vi "ExportToWord.vi"(11 "DataForAnalysis":T1(array[cluster]) {"Eff" scale=0.0..30.0; "JVmetrics" format="%#_4g"}) -> ()   [LabVIEW 2020]
uses:
  <vilib>/Utility/NIReport.llb/NI_report.lvclass
  <vilib>/addons/_office/word.llb/Word Easy Table (num).vi
  <vilib>/Utility/NIReport.llb/Append Report Text (str wrap).vi
  <vilib>/addons/_office/_exclsub.llb/font.ctl
panel:
  in  "Plot Color 2":u32[](array[colorbox])=[16711686]
  in  "Plot Area Color 2":u32(colorbox)=16777215
  in  "Axis Font 2":T2={"font style"="", "bold"=FALSE, "italic"=FALSE, "underline"=FALSE, "size"=10.0, "color"=4278190080} {"size" format="%.2f"}
  in  "Y Axis Configuration 2":T3={"Autoscale"=TRUE, "min"=0.0, "max"=0.0, "scale type"=-4132} {"scale type" items=["xlScaleLinear"=-4132, "xlScaleLogarithmic"=-4133]; "max" format="%.2f"; "min" format="%.2f"}
  in  "X Axis Configuration 2":T4={"autoscale"=TRUE, "min"=0.0, "max"=0.0, "scale type"=-4132} {"scale type" items=["xlScaleLinear"=-4132, "xlScaleLogarithmic"=-4133]; "max" format="%.2f"; "min" format="%.2f"}
  in  "graph title (\"\") 2":string="Transient data"
  in  "yAxisT 2":string="Power (mW/cm2)"
  in  "XAxisT 2":string="time (s)"
  out "transposed array":dbl[][](array[numeric])=[[1.0, 0.0], [0.0, 0.0], [0.0, 0.0], [1.0, 0.0], [0.0, 0.0], [1.0, 1.0]]
  in  "column headers":string[](array[string])=["1st scan", "2nd scan"]
  in  "indent and spacing":T5 {"at" format="%.2f"; "after" format="%.2f"; "before" format="%.2f"; "by" format="%.2f"; "right" format="%.2f"; "left" format="%.2f"}
  in  "line and page breaks":T6={"widow/orphan ctrl"=2, "Keeps lines together"=0, "keep with next"=0, "page break before"=0, "suppress line numbers"=0, "don't hyphenate"=0} {"don't hyphenate" items=["Unchanged", "No", "Yes"]; "suppress line numbers" items=["Unchanged", "No", "Yes"]; "page break before" items=["Unchanged", "No", "Yes"]; "keep with next" items=["Unchanged", "No", "Yes"]; "Keeps lines together" items=["Unchanged", "No", "Yes"]; "widow/orphan ctrl" items=["Unchanged", "No", "Yes"]}
  in  "auto format (none)":i32=-1
  in  "font":T7={"font name"="", "font size"=10.0, "bold"=2, "italic"=0, "underline"=0, "strike through"=0, "font color"=16777216} {"font size" format="%0.2f"; "strike through" items=["Unchanged", "Yes", "No"]; "underline" items=["Unchanged", "Yes", "No"]; "italic" items=["Unchanged", "Yes", "No"]; "bold" items=["Unchanged", "Yes", "No"]}
  in  "HeaderJVMetrics":string[](array[string])=["Voc (V)", "Jsc (mA/cm2)", "FF", "P (mW/cm2)", "Hyst P1/P2", "scan rate (mV/s)", "intensity (suns)", "temperature (C)"]
  in  "XAxisT":string="Voltage (V)"
  in  "yAxisT":string="Current Density (mA/cm2)"
  in  "graph title (\"\")":string="JV data"
  in  "X Axis Configuration":T4={"autoscale"=TRUE, "min"=0.0, "max"=0.0, "scale type"=-4132} {"scale type" items=["xlScaleLinear"=-4132, "xlScaleLogarithmic"=-4133]; "max" format="%.2f"; "min" format="%.2f"}
  in  "Y Axis Configuration":T3={"Autoscale"=TRUE, "min"=0.0, "max"=0.0, "scale type"=-4132} {"scale type" items=["xlScaleLinear"=-4132, "xlScaleLogarithmic"=-4133]; "max" format="%.2f"; "min" format="%.2f"}
  in  "Axis Font":T2={"font style"="", "bold"=FALSE, "italic"=FALSE, "underline"=FALSE, "size"=10.0, "color"=4278190080} {"size" format="%.2f"}
  in  "Plot Area Color":u32(colorbox)=16777215
  in  "Plot Color":u32[](array[colorbox])=[16860]
  # "indentation"
  # "spacing"
  # "pagination"
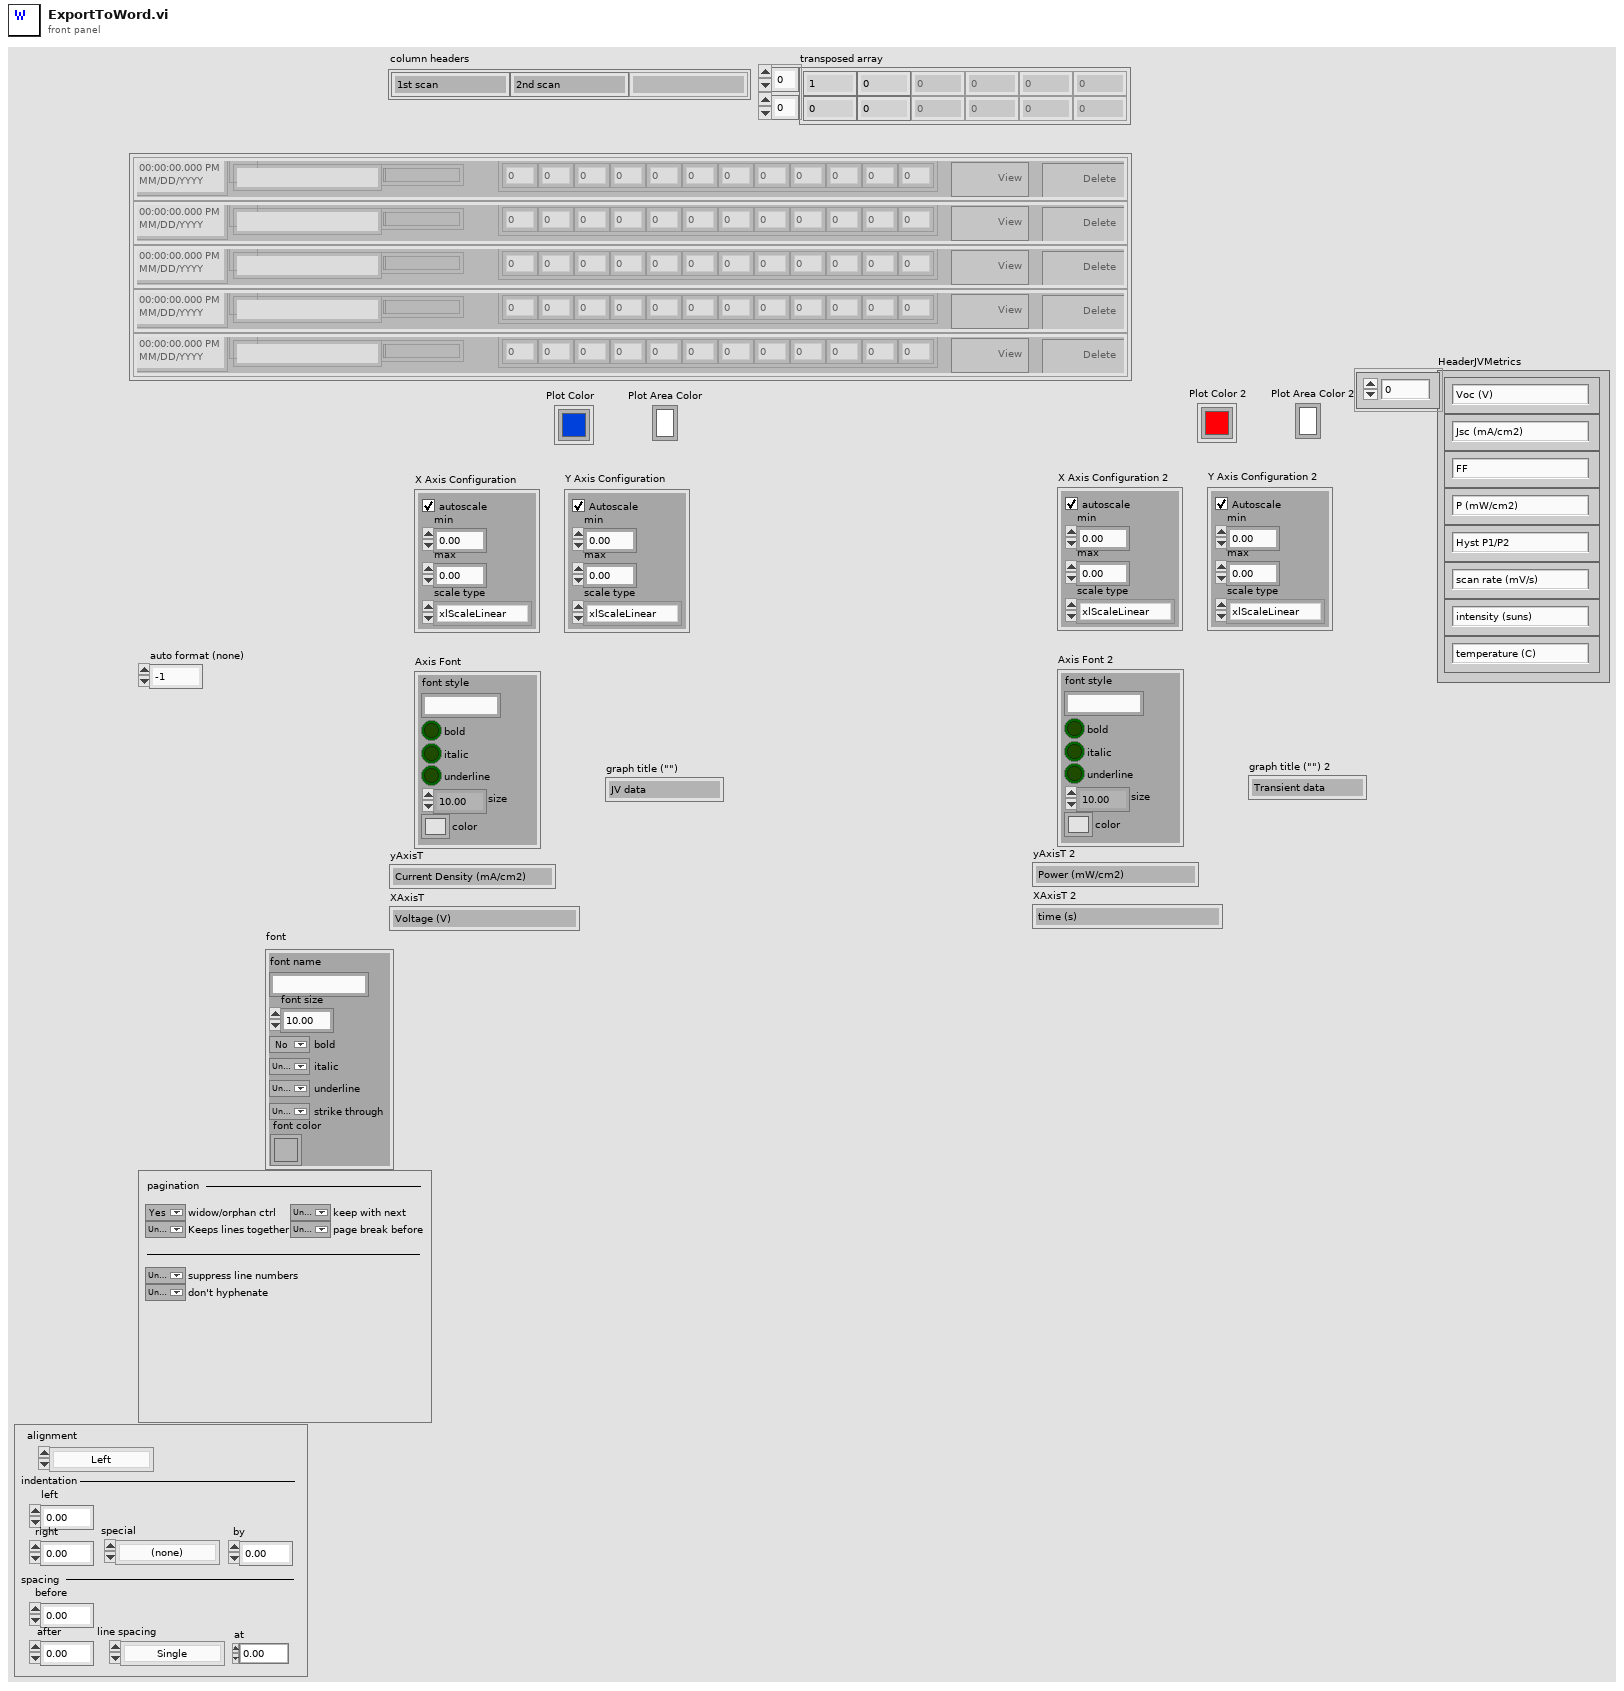
[diagram p1: front panel]
types:
  T1 = cluster{"JVData":dbl[][], "JVmetrics":dbl[], "TransientData":dbl[][], "TimeMeasured":timestamp, "Name":string, "Delete":bool, "Eff":u8, "ViewJV":bool}[]
  T2 = cluster{"font style":string, "bold":bool, "italic":bool, "underline":bool, "size":sgl, "color":u32}
  T3 = cluster{"Autoscale":bool, "min":dbl, "max":dbl, "scale type":i32}
  T4 = cluster{"autoscale":bool, "min":dbl, "max":dbl, "scale type":i32}
  T5 = cluster{"alignment":enum16{"Left", "Centered", "Right", "Justify"}, "left":dbl, "right":dbl, "special":enum16{"(none)", "First line", "Hanging"}, "by":dbl, "before":dbl, "after":dbl, "line spacing":enum16{"Single", "1,5 lines", "Double", "At least", "Exactly", "Multiple"}, "at":dbl}
  T6 = cluster{"widow/orphan ctrl":u16, "Keeps lines together":u16, "keep with next":u16, "page break before":u16, "suppress line numbers":u16, "don't hyphenate":u16}
  T7 = typedef "NI_ReportGenerationToolkit.lvlib/font.ctl" = cluster{"font name":string, "font size":dbl, "bold":u16, "italic":u16, "underline":u16, "strike through":u16, "font color":u32}
  T8 = enum16{"Standard Report", "HTML", "Word", "Excel"}
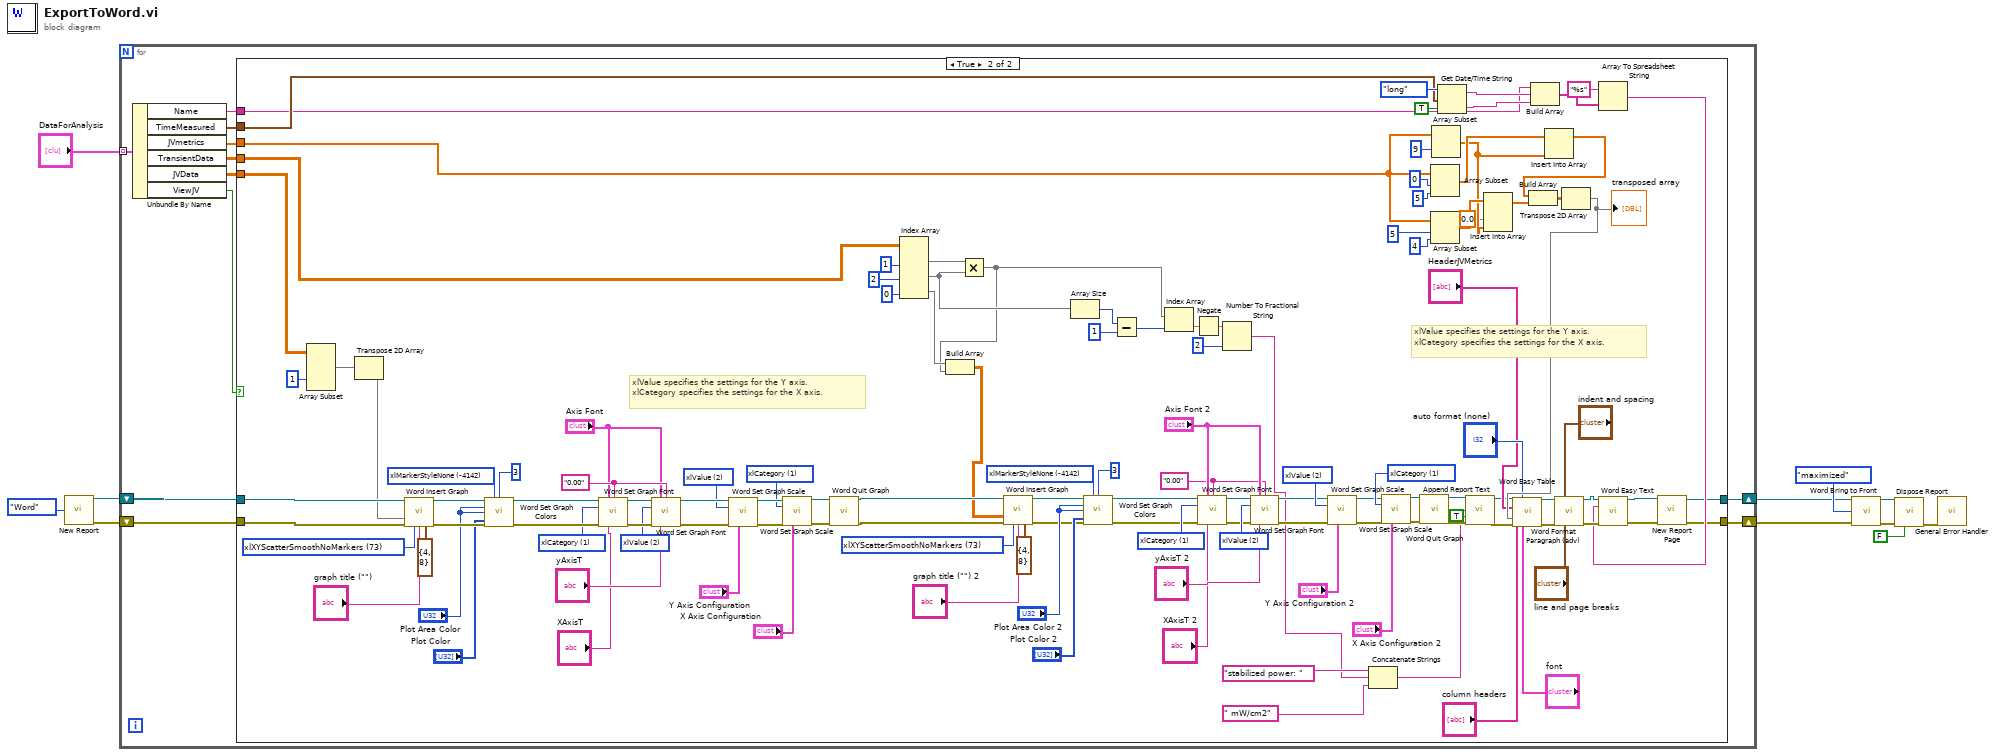
[diagram p0: block diagram]
diagram:
  n1 = call <vilib>:"New Report.vi"("report type"=T8."Word") -> ("report out"=w10:refnum<class "NI_report.lvclass">, "error out"=w11:errorcluster)  [unwired: 13 in]
  n2 = for {
    shift-right: [w17] -> w3
    shift-left: w11 -> [w22]
    shift-right: [w16] -> w2
    shift-left: w10 -> [w21]
    tunnel: "DataForAnalysis" -> [w15] mode=indexing
    n3 = Unbundle By Name(w15) -> ("Name"=w19:string, "TimeMeasured"=w20:timestamp, "JVmetrics"=w18:dbl[], "TransientData"=w13:dbl[][], "JVData"=w14:dbl[][], "ViewJV"=w12:bool)
    n4 = case shown="True" w12 {
      tunnel: w22 -> [w23 w151]
      tunnel: w21 -> [w24 w150]
      tunnel: w20 -> [_ w119]
      tunnel: w19 -> [_ w104]
      tunnel: w18 -> [_ w98]
      tunnel: [w23 w60] -> w17
      tunnel: [w24 w59] -> w16
      tunnel: w14 -> [_ w35]
      tunnel: w13 -> [_ w40]
      frame False {
      }
      frame True {
        w89 = "0.00" ("number format (general)")
        w86 = 1 items=["xlCategory"=1, "xlSeriesAxis"=3, "xlValue"=2] ("axis type")
        w83 = 2 items=["xlCategory"=1, "xlSeriesAxis"=3, "xlValue"=2] ("axis type")
        w80 = 2 items=["xlCategory"=1, "xlSeriesAxis"=3, "xlValue"=2] ("axis type")
        w77 = 1 items=["xlCategory"=1, "xlSeriesAxis"=3, "xlValue"=2] ("axis type")
        w74 = -4142 items=["xlMarkerStyleAutomatic"=-4105, "xlMarkerStyleCircle"=8, "xlMarkerStyleDash"=-4115, "xlMarkerStyleDiamond"=2, "xlMarkerStyleDot"=-4118, "xlMarkerStyleNone"=-4142, "xlMarkerStylePicture"=-4147, "xlMarkerStylePlus"=9, "xlMarkerStyleSquare"=1, "xlMarkerStyleStar"=5, "xlMarkerStyleTriangle"=3, "xlMarkerStyleX"=-4168] ("marker style")
        w69 = 73 items=["xlColumnClustered"=51, "xlColumnStacked"=52, "xlColumnStacked100"=53, "xl3DColumnClustered"=54, "xl3DColumnStacked"=55, "xl3DColumnStacked100"=56, "xlBarClustered"=57, "xlBarStacked"=58, "xlBarStacked100"=59, "xl3DBarClustered"=60, "xl3DBarStacked"=61, "xl3DBarStacked100"=62, "xlLineStacked"=63, "xlLineStacked100"=64, "xlLineMarkers"=65, "xlLineMarkersStacked"=66, "xlLineMarkersStacked100"=67, "xlPieOfPie"=68, "xlPieExploded"=69, "xl3DPieExploded"=70, "xlBarOfPie"=71, "xlXYScatterSmooth"=72, "xlXYScatterSmoothNoMarkers"=73, "xlXYScatterLines"=74, "xlXYScatterLinesNoMarkers"=75, "xlAreaStacked"=76, "xlAreaStacked100"=77, "xl3DAreaStacked"=78, "xl3DAreaStacked100"=79, "xlDoughnutExploded"=80, "xlRadarMarkers"=81, "xlRadarFilled"=82, "xlSurface"=83, "xlSurfaceWireframe"=84, "xlSurfaceTopView"=85, "xlSurfaceTopViewWireframe"=86, "xlBubble"=15, "xlBubble3DEffect"=87, "xlStockHLC"=88, "xlStockOHLC"=89, "xlStockVHLC"=90, "xlStockVOHLC"=91, "xlCylinderColClustered"=92, "xlCylinderColStacked"=93, "xlCylinderColStacked100"=94, "xlCylinderBarClustered"=95, "xlCylinderBarStacked"=96, "xlCylinderBarStacked100"=97, "xlCylinderCol"=98, "xlConeColClustered"=99, "xlConeColStacked"=100, "xlConeColStacked100"=101, "xlConeBarClustered"=102, "xlConeBarStacked"=103, "xlConeBarStacked100"=104, "xlConeCol"=105, "xlPyramidColClustered"=106, "xlPyramidColStacked"=107, "xlPyramidColStacked100"=108, "xlPyramidBarClustered"=109, "xlPyramidBarStacked"=110, "xlPyramidBarStacked100"=111, "xlPyramidCol"=112, "xl3DColumn"=-4100, "xlLine"=4, "xl3DLine"=-4101, "xl3DPie"=-4102, "xlPie"=5, "xlXYScatter"=-4169, "xl3DArea"=-4098, "xlArea"=1, "xlDoughnut"=-4120, "xlRadar"=-4151] ("chart type")
        w129 = "0.00" ("number format (general)")
        w132 = 1 items=["xlCategory"=1, "xlSeriesAxis"=3, "xlValue"=2] ("axis type")
        w135 = 2 items=["xlCategory"=1, "xlSeriesAxis"=3, "xlValue"=2] ("axis type")
        w138 = 2 items=["xlCategory"=1, "xlSeriesAxis"=3, "xlValue"=2] ("axis type")
        w141 = 1 items=["xlCategory"=1, "xlSeriesAxis"=3, "xlValue"=2] ("axis type")
        w144 = -4142 items=["xlMarkerStyleAutomatic"=-4105, "xlMarkerStyleCircle"=8, "xlMarkerStyleDash"=-4115, "xlMarkerStyleDiamond"=2, "xlMarkerStyleDot"=-4118, "xlMarkerStyleNone"=-4142, "xlMarkerStylePicture"=-4147, "xlMarkerStylePlus"=9, "xlMarkerStyleSquare"=1, "xlMarkerStyleStar"=5, "xlMarkerStyleTriangle"=3, "xlMarkerStyleX"=-4168] ("marker style")
        w149 = 73 items=["xlColumnClustered"=51, "xlColumnStacked"=52, "xlColumnStacked100"=53, "xl3DColumnClustered"=54, "xl3DColumnStacked"=55, "xl3DColumnStacked100"=56, "xlBarClustered"=57, "xlBarStacked"=58, "xlBarStacked100"=59, "xl3DBarClustered"=60, "xl3DBarStacked"=61, "xl3DBarStacked100"=62, "xlLineStacked"=63, "xlLineStacked100"=64, "xlLineMarkers"=65, "xlLineMarkersStacked"=66, "xlLineMarkersStacked100"=67, "xlPieOfPie"=68, "xlPieExploded"=69, "xl3DPieExploded"=70, "xlBarOfPie"=71, "xlXYScatterSmooth"=72, "xlXYScatterSmoothNoMarkers"=73, "xlXYScatterLines"=74, "xlXYScatterLinesNoMarkers"=75, "xlAreaStacked"=76, "xlAreaStacked100"=77, "xl3DAreaStacked"=78, "xl3DAreaStacked100"=79, "xlDoughnutExploded"=80, "xlRadarMarkers"=81, "xlRadarFilled"=82, "xlSurface"=83, "xlSurfaceWireframe"=84, "xlSurfaceTopView"=85, "xlSurfaceTopViewWireframe"=86, "xlBubble"=15, "xlBubble3DEffect"=87, "xlStockHLC"=88, "xlStockOHLC"=89, "xlStockVHLC"=90, "xlStockVOHLC"=91, "xlCylinderColClustered"=92, "xlCylinderColStacked"=93, "xlCylinderColStacked100"=94, "xlCylinderBarClustered"=95, "xlCylinderBarStacked"=96, "xlCylinderBarStacked100"=97, "xlCylinderCol"=98, "xlConeColClustered"=99, "xlConeColStacked"=100, "xlConeColStacked100"=101, "xlConeBarClustered"=102, "xlConeBarStacked"=103, "xlConeBarStacked100"=104, "xlConeCol"=105, "xlPyramidColClustered"=106, "xlPyramidColStacked"=107, "xlPyramidColStacked100"=108, "xlPyramidBarClustered"=109, "xlPyramidBarStacked"=110, "xlPyramidBarStacked100"=111, "xlPyramidCol"=112, "xl3DColumn"=-4100, "xlLine"=4, "xl3DLine"=-4101, "xl3DPie"=-4102, "xlPie"=5, "xlXYScatter"=-4169, "xl3DArea"=-4098, "xlArea"=1, "xlDoughnut"=-4120, "xlRadar"=-4151] ("chart type")
        # "xlValue specifies the settings for the Y axis. xlCategory specifies the settings for the X axis."
        # "xlValue specifies the settings for the Y axis. xlCategory specifies the settings for the X axis."
        n5 = Array Subset(array=w35, index (col)=1 ("index")) -> (w32:dbl[][])  [unwired: 3 in]
        n6 = Transpose 2D Array(2D array=w32) -> (transposed array=w33:dbl[][])
        n7 = call <vilib>:"Word Insert Graph.vi"("report in"=w150, "data"=w33, "error in (no error)"=w151, "graph type (col clustered)"=w149, "graph title (\"\")"="graph title (\"\")", "graph size (5, 5)"=cluster{"Height":i32, "Width":i32} {"Height"=4, "Width"=8} ("chart size")) -> ("report out"=w146:refnum<class "NI_report.lvclass">, "error out"=w147:errorcluster)  [unwired: 6 in, 2 out]
        n8 = call <vilib>:"Word Set Graph Colors.vi"("report in"=w146, "marker style (none)"=w144, "weight (1)"=i16 3 ("weight"), "plot area color (w)"="Plot Area Color", "graph area color (w)"="Plot Area Color", "error in (no error)"=w147, "plot colors"="Plot Color") -> ("report out"=w142:refnum<class "NI_report.lvclass">, "error out"=w143:errorcluster)  [unwired: 7 in]
        n9 = call <vilib>:"Word Set Graph Font.vi"("report in"=w142, "axis font"="Axis Font", "number format (general)"=w129, "axis type (category)"=w141, "error in (no error)"=w143, "title (\"\")"="XAxisT") -> ("report out"=w139:refnum<class "NI_report.lvclass">, "error out"=w140:errorcluster)  [unwired: 8 in]
        n10 = call <vilib>:"Word Set Graph Font.vi"("report in"=w139, "axis font"="Axis Font", "number format (general)"=w129, "axis type (category)"=w138, "error in (no error)"=w140, "title (\"\")"="yAxisT") -> ("report out"=w136:refnum<class "NI_report.lvclass">, "error out"=w137:errorcluster)  [unwired: 8 in]
        n11 = call <vilib>:"Word Set Graph Scale.vi"("report in"=w136, "axis type (xlCategory)"=w135, "error in (no error)"=w137, "axis config"="Y Axis Configuration") -> ("report out"=w133:refnum<class "NI_report.lvclass">, "error out"=w134:errorcluster)  [unwired: 10 in]
        n12 = call <vilib>:"Word Set Graph Scale.vi"("report in"=w133, "axis type (xlCategory)"=w132, "error in (no error)"=w134, "axis config"="X Axis Configuration") -> ("report out"=w131:refnum<class "NI_report.lvclass">, "error out"=w130:errorcluster)  [unwired: 10 in]
        n13 = call <vilib>:"Word Quit Graph.vi"("report in"=w131, "error in (no error)"=w130) -> ("report out"=w68:refnum<class "NI_report.lvclass">, "error out"=w67:errorcluster)  [unwired: 12 in]
        n14 = Index Array(array=w40, index (col) #1=1 ("disabled index (col)"), index (col) #2=2 ("index (col)"), index (col) #3=0 ("index (col)")) -> (element #1=w44:dbl[], element #2=w43:dbl[], element #3=w38:dbl[])  [unwired: 3 in]
        n15 = Multiply(x=w44, y=w43) -> (x*y=w37:dbl[])
        n16 = Build Array(w38, w37) -> (w36:dbl[][])
        n17 = call <vilib>:"Word Insert Graph.vi"("report in"=w68, "data"=w36, "error in (no error)"=w67, "graph type (col clustered)"=w69, "graph title (\"\")"="graph title (\"\") 2", "graph size (5, 5)"=cluster{"Height":i32, "Width":i32} {"Height"=4, "Width"=8} ("chart size")) -> ("report out"=w72:refnum<class "NI_report.lvclass">, "error out"=w71:errorcluster)  [unwired: 6 in, 2 out]
        n18 = Array Size(array=w43) -> (size(s)=w48:i32)
        n19 = call <vilib>:"Word Set Graph Colors.vi"("report in"=w72, "marker style (none)"=w74, "weight (1)"=i16 3 ("weight"), "plot area color (w)"="Plot Area Color 2", "graph area color (w)"="Plot Area Color 2", "error in (no error)"=w71, "plot colors"="Plot Color 2") -> ("report out"=w76:refnum<class "NI_report.lvclass">, "error out"=w75:errorcluster)  [unwired: 7 in]
        n20 = Subtract(x=w48, y=1) -> (x-y=w49:i32)
        n21 = Index Array(array=w37, index=w49) -> (element=w30:dbl)
        n22 = Negate(x=w30) -> (-x=w31:dbl)
        n23 = call <vilib>:"Word Set Graph Font.vi"("report in"=w76, "axis font"="Axis Font 2", "number format (general)"=w89, "axis type (category)"=w77, "error in (no error)"=w75, "title (\"\")"="XAxisT 2") -> ("report out"=w79:refnum<class "NI_report.lvclass">, "error out"=w78:errorcluster)  [unwired: 8 in]
        n24 = Number To Fractional String(number=w31, precision (6)=i16 2) -> (F-format string=w42:string)  [unwired: 2 in]
        n25 = call <vilib>:"Word Set Graph Font.vi"("report in"=w79, "axis font"="Axis Font 2", "number format (general)"=w89, "axis type (category)"=w80, "error in (no error)"=w78, "title (\"\")"="yAxisT 2") -> ("report out"=w82:refnum<class "NI_report.lvclass">, "error out"=w81:errorcluster)  [unwired: 8 in]
        n26 = call <vilib>:"Word Set Graph Scale.vi"("report in"=w82, "axis type (xlCategory)"=w83, "error in (no error)"=w81, "axis config"="Y Axis Configuration 2") -> ("report out"=w85:refnum<class "NI_report.lvclass">, "error out"=w84:errorcluster)  [unwired: 10 in]
        n27 = Concatenate Strings("stabilized power: ", w42, " mW/cm2") -> (w52:string)
        n28 = call <vilib>:"Word Set Graph Scale.vi"("report in"=w85, "axis type (xlCategory)"=w86, "error in (no error)"=w84, "axis config"="X Axis Configuration 2") -> ("report out"=w87:refnum<class "NI_report.lvclass">, "error out"=w88:errorcluster)  [unwired: 10 in]
        n29 = call <vilib>:"Word Quit Graph.vi"("report in"=w87, "error in (no error)"=w88) -> ("report out"=w57:refnum<class "NI_report.lvclass">, "error out"=w54:errorcluster)  [unwired: 12 in]
        n30 = Array Subset(array=w98, index=0, length=5) -> (w97:dbl[])
        n31 = Array Subset(array=w98, index=5 ("length"), length=4) -> (w27:dbl[])
        n32 = Array Subset(array=w98, index=9 ("length")) -> (w26:dbl[])  [unwired: 1 in]
        n33 = Get Date/Time String(date format (0)=enum16{"short", "long", "abbreviated"}."long", seconds (now)=w119, want seconds? (F)=TRUE) -> (date string=w118:string, time string=w120:string)
        n34 = call-poly <vilib>:"Append Report Text.vi"("report in"=w57, "text"=w52, "append on new line? (F)"=TRUE, "error in (no error)"=w54) -> ("report out"=w56:refnum<class "NI_report.lvclass">, "error out"=w55:errorcluster)  [unwired: 8 in, 2 out]
        n35 = Insert Into Array(array=w27, new element #1=0.0 ("new element/subarray"), new element #2=w26) -> (w28:dbl[])  [unwired: 1 in]
        n36 = Build Array(w104, w118, w120) -> (w103:string[])
        n37 = Insert Into Array(array=w97, new element=w26) -> (w96:dbl[])  [unwired: 1 in]
        n38 = Build Array(w96, w28) -> (w109:dbl[][])
        n39 = Transpose 2D Array(2D array=w109) -> (transposed array=w117:dbl[][])
        "transposed array" <- w117
        n40 = call-poly <vilib>:"Word Easy Table.vi"("report in"=w56, "auto format (none)"="auto format (none)", "row headers"="HeaderJVMetrics", "column headers"="column headers", "text data"=w117, "error in (no error)"=w55, "font"="font") -> ("report out"=w114:refnum<class "NI_report.lvclass">, "error out"=w111:errorcluster)  [unwired: 6 in, 1 out]
        n41 = call <vilib>:"Word Format Paragraph (adv).vi"("report in"=w114, "indent and spacing"="indent and spacing", "error in (no error)"=w111, "line and page breaks"="line and page breaks") -> ("report out"=w107:refnum<class "NI_report.lvclass">, "error out"=w106:errorcluster)  [unwired: 10 in]
        n42 = Array To Spreadsheet String(array=w103, 3:"%s" ("format string")) -> (spreadsheet string=w102:string)  [unwired: 1 in]
        n43 = call <vilib>:"Word Easy Text.vi"("report in"=w107, "text"=w102, "error in (no error)"=w106) -> ("report out"=w62:refnum<class "NI_report.lvclass">, "error out"=w61:errorcluster)  [unwired: 10 in, 1 out]
        n44 = call-dynamic "New Report Page.vi"("report in"=w62, "error in (no error)"=w61) -> ("report out"=w59:refnum<class "NI_report.lvclass">, "error out"=w60:errorcluster)  [unwired: 12 in]
      }
    }
  }
  n45 = call <vilib>:"Word Bring to Front.vi"("report in"=w2, "window state (maximized)"=enum16{"maximized", "minimized", "normal"}."maximized", "error in (no error)"=w3) -> ("report out"=w7:refnum<class "NI_report.lvclass">, "error out"=w6:errorcluster)  [unwired: 11 in]
  n46 = call-dynamic "Dispose Report.vi"("report in"=w7, "error in (no error)"=w6, "close report? (T)"=FALSE ("Close Report? (T)")) -> ("error out"=w5:errorcluster)  [unwired: 12 in]
  n47 = call <vilib>:"General Error Handler.vi"("error in (no error)"=w5) -> ()  [unwired: 10 in, 5 out]
